vi "Convert String Data Type.vi"(5 "src byte order":T1(ring), 7 "dst byte order":T1(ring), 8 "error in (no error)":errorcluster, 9 "dst data type":T2, 10 "src data type":T2, 11 "src data in":string) -> (0 "error out":errorcluster, 3 "dst data out":string)   [LabVIEW 2019, in "DSF Core.lvlib" / "Buffer Converter.lvclass"]
uses:
  Buffer Converter.lvclass
  Typedefs/DSF Data Type.ctl
  DSF Core.lvlib
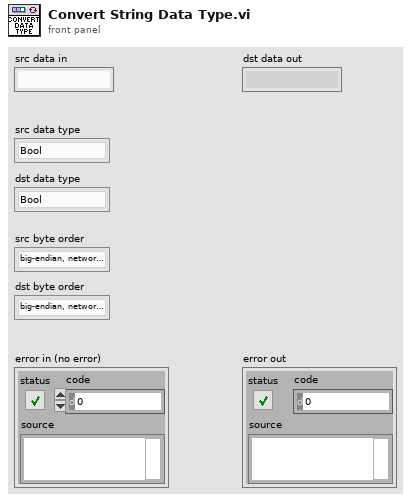
[diagram p1: front panel]
types:
  T1 = enum16{"big-endian, network order", "native, host order", "little-endian"}
  T2 = typedef "DSF Core.lvlib/DSF Data Type.ctl" = enum8{"Bool", "SGL", "DBL", "I8", "I16", "I32", "I64", "U8", "U16", "U32", "U64"}
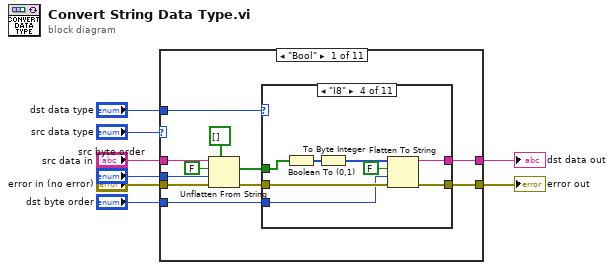
[diagram p0: block diagram]
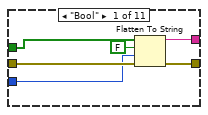
[diagram p2: hidden frame]
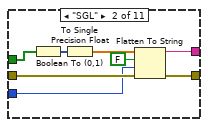
[diagram p3: hidden frame]
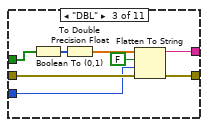
[diagram p4: hidden frame]
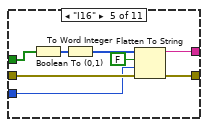
[diagram p5: hidden frame]
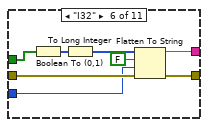
[diagram p6: hidden frame]
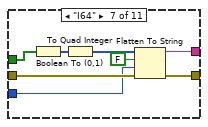
[diagram p7: hidden frame]
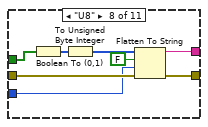
[diagram p8: hidden frame]
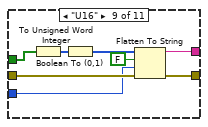
[diagram p9: hidden frame]
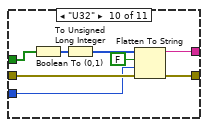
[diagram p10: hidden frame]
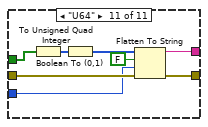
[diagram p11: hidden frame]
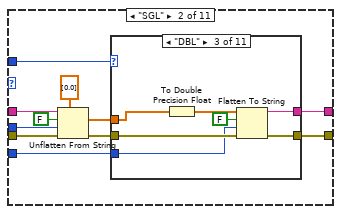
[diagram p12: hidden frame]
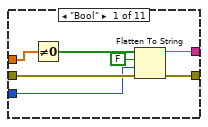
[diagram p13: hidden frame]
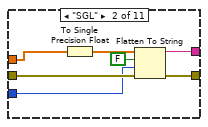
[diagram p14: hidden frame]
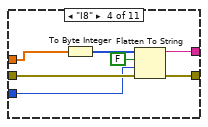
[diagram p15: hidden frame]
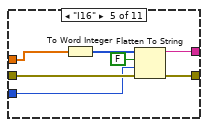
[diagram p16: hidden frame]
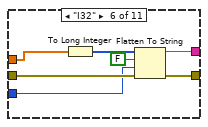
[diagram p17: hidden frame]
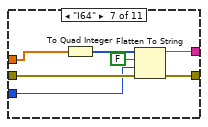
[diagram p18: hidden frame]
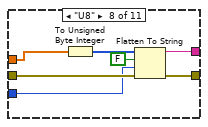
[diagram p19: hidden frame]
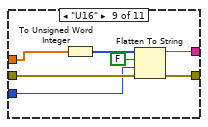
[diagram p20: hidden frame]
diagram:
  n1 = case shown="\"Bool\"" "src data type" {
    tunnel: "src data in" -> [w17 w114 w202 w290 w378 w466 w554 w642 w730 w818 w906]
    tunnel: "error in (no error)" -> [w16 w113 w201 w289 w377 w465 w553 w641 w729 w817 w905]
    tunnel: "dst data type" -> [w15 w112 w200 w288 w376 w464 w552 w640 w728 w816 w904]
    tunnel: [w12 w109 w197 w285 w373 w461 w549 w637 w725 w813 w901] -> w2
    tunnel: [w11 w108 w196 w284 w372 w460 w548 w636 w724 w812 w900] -> w8
    tunnel: "src byte order" -> [w10 w107 w195 w283 w371 w459 w547 w635 w723 w811 w899]
    tunnel: "dst byte order" -> [w9 w106 w194 w282 w370 w458 w546 w634 w722 w810 w898]
    frame "Bool" {
      n2 = Unflatten From String(type=bool[] [], binary string=w17, data includes array or string size? (T)=FALSE, byte order (0:big-endian, network order)=w10, error in (no error)=w16) -> (value=w14:bool[], error out=w13:errorcluster)  [unwired: 1 out]
      n3 = case shown="\"I8\"" w15 {
        tunnel: w14 -> [w25 w33 w41 w49 w57 w65 w73 w81 w89 w97 w105]
        tunnel: w13 -> [w24 w32 w40 w48 w56 w64 w72 w80 w88 w96 w104]
        tunnel: [w23 w31 w39 w47 w55 w63 w71 w79 w87 w95 w103] -> w12
        tunnel: [w22 w30 w38 w46 w54 w62 w70 w78 w86 w94 w102] -> w11
        tunnel: w9 -> [w21 w29 w37 w45 w53 w61 w69 w77 w85 w93 w101]
        frame "Bool" {
          n4 = Flatten To String(anything=w25, prepend array or string size? (T)=FALSE, byte order (0:big-endian, network order)=w21, error in (no error)=w24) -> (data string=w22:string, error out=w23:errorcluster)  [unwired: 1 out]
        }
        frame "SGL" {
          n5 = Boolean To (0,1)(Boolean=w33) -> (0, 1=w26:i16[])
          n6 = To Single Precision Float(number=w26) -> (single precision float=w27:sgl[])
          n7 = Flatten To String(anything=w27, prepend array or string size? (T)=FALSE, byte order (0:big-endian, network order)=w29, error in (no error)=w32) -> (data string=w30:string, error out=w31:errorcluster)  [unwired: 1 out]
        }
        frame "DBL" {
          n8 = Boolean To (0,1)(Boolean=w41) -> (0, 1=w34:i16[])
          n9 = To Double Precision Float(number=w34) -> (double precision float=w35:dbl[])
          n10 = Flatten To String(anything=w35, prepend array or string size? (T)=FALSE, byte order (0:big-endian, network order)=w37, error in (no error)=w40) -> (data string=w38:string, error out=w39:errorcluster)  [unwired: 1 out]
        }
        frame "I8" {
          n11 = Boolean To (0,1)(Boolean=w49) -> (0, 1=w42:i16[])
          n12 = To Byte Integer(number=w42) -> (8bit integer=w43:i8[])
          n13 = Flatten To String(anything=w43, prepend array or string size? (T)=FALSE, byte order (0:big-endian, network order)=w45, error in (no error)=w48) -> (data string=w46:string, error out=w47:errorcluster)  [unwired: 1 out]
        }
        frame "I16" {
          n14 = Boolean To (0,1)(Boolean=w57) -> (0, 1=w50:i16[])
          n15 = To Word Integer(number=w50) -> (16bit integer=w51:i16[])
          n16 = Flatten To String(anything=w51, prepend array or string size? (T)=FALSE, byte order (0:big-endian, network order)=w53, error in (no error)=w56) -> (data string=w54:string, error out=w55:errorcluster)  [unwired: 1 out]
        }
        frame "I32" {
          n17 = Boolean To (0,1)(Boolean=w65) -> (0, 1=w58:i16[])
          n18 = To Long Integer(number=w58) -> (32bit integer=w59:i32[])
          n19 = Flatten To String(anything=w59, prepend array or string size? (T)=FALSE, byte order (0:big-endian, network order)=w61, error in (no error)=w64) -> (data string=w62:string, error out=w63:errorcluster)  [unwired: 1 out]
        }
        frame "I64" {
          n20 = Boolean To (0,1)(Boolean=w73) -> (0, 1=w66:i16[])
          n21 = To Quad Integer(1:w66) -> (0:w67:i64[])
          n22 = Flatten To String(anything=w67, prepend array or string size? (T)=FALSE, byte order (0:big-endian, network order)=w69, error in (no error)=w72) -> (data string=w70:string, error out=w71:errorcluster)  [unwired: 1 out]
        }
        frame "U8" {
          n23 = Boolean To (0,1)(Boolean=w81) -> (0, 1=w74:i16[])
          n24 = To Unsigned Byte Integer(number=w74) -> (unsigned 8bit integer=w75:u8[])
          n25 = Flatten To String(anything=w75, prepend array or string size? (T)=FALSE, byte order (0:big-endian, network order)=w77, error in (no error)=w80) -> (data string=w78:string, error out=w79:errorcluster)  [unwired: 1 out]
        }
        frame "U16" {
          n26 = Boolean To (0,1)(Boolean=w89) -> (0, 1=w82:i16[])
          n27 = To Unsigned Word Integer(number=w82) -> (unsigned 16bit integer=w83:u16[])
          n28 = Flatten To String(anything=w83, prepend array or string size? (T)=FALSE, byte order (0:big-endian, network order)=w85, error in (no error)=w88) -> (data string=w86:string, error out=w87:errorcluster)  [unwired: 1 out]
        }
        frame "U32" {
          n29 = Boolean To (0,1)(Boolean=w97) -> (0, 1=w90:i16[])
          n30 = To Unsigned Long Integer(number=w90) -> (unsigned 32bit integer=w91:u32[])
          n31 = Flatten To String(anything=w91, prepend array or string size? (T)=FALSE, byte order (0:big-endian, network order)=w93, error in (no error)=w96) -> (data string=w94:string, error out=w95:errorcluster)  [unwired: 1 out]
        }
        frame "U64" {
          n32 = Boolean To (0,1)(Boolean=w105) -> (0, 1=w98:i16[])
          n33 = To Unsigned Quad Integer(1:w98) -> (0:w99:u64[])
          n34 = Flatten To String(anything=w99, prepend array or string size? (T)=FALSE, byte order (0:big-endian, network order)=w101, error in (no error)=w104) -> (data string=w102:string, error out=w103:errorcluster)  [unwired: 1 out]
        }
      }
    }
    frame "SGL" {
      n35 = Unflatten From String(type=sgl[] [0.0], binary string=w114, data includes array or string size? (T)=FALSE, byte order (0:big-endian, network order)=w107, error in (no error)=w113) -> (value=w111:sgl[], error out=w110:errorcluster)  [unwired: 1 out]
      n36 = case shown="\"DBL\"" w112 {
        tunnel: w111 -> [w118 w125 w132 w139 w146 w153 w160 w167 w174 w181 w188]
        tunnel: w110 -> [w123 w130 w137 w144 w151 w158 w165 w172 w179 w186 w193]
        tunnel: [w122 w129 w136 w143 w150 w157 w164 w171 w178 w185 w192] -> w109
        tunnel: [w121 w128 w135 w142 w149 w156 w163 w170 w177 w184 w191] -> w108
        tunnel: w106 -> [w120 w127 w134 w141 w148 w155 w162 w169 w176 w183 w190]
        frame "Bool" {
          n37 = Not Equal To 0?(x=w118) -> (x != 0?=w117:bool[])
          n38 = Flatten To String(anything=w117, prepend array or string size? (T)=FALSE, byte order (0:big-endian, network order)=w120, error in (no error)=w123) -> (data string=w121:string, error out=w122:errorcluster)  [unwired: 1 out]
        }
        frame "SGL" {
          n39 = To Single Precision Float(number=w125) -> (single precision float=w124:sgl[])
          n40 = Flatten To String(anything=w124, prepend array or string size? (T)=FALSE, byte order (0:big-endian, network order)=w127, error in (no error)=w130) -> (data string=w128:string, error out=w129:errorcluster)  [unwired: 1 out]
        }
        frame "DBL" {
          n41 = To Double Precision Float(number=w132) -> (double precision float=w131:dbl[])
          n42 = Flatten To String(anything=w131, prepend array or string size? (T)=FALSE, byte order (0:big-endian, network order)=w134, error in (no error)=w137) -> (data string=w135:string, error out=w136:errorcluster)  [unwired: 1 out]
        }
        frame "I8" {
          n43 = To Byte Integer(number=w139) -> (8bit integer=w138:i8[])
          n44 = Flatten To String(anything=w138, prepend array or string size? (T)=FALSE, byte order (0:big-endian, network order)=w141, error in (no error)=w144) -> (data string=w142:string, error out=w143:errorcluster)  [unwired: 1 out]
        }
        frame "I16" {
          n45 = To Word Integer(number=w146) -> (16bit integer=w145:i16[])
          n46 = Flatten To String(anything=w145, prepend array or string size? (T)=FALSE, byte order (0:big-endian, network order)=w148, error in (no error)=w151) -> (data string=w149:string, error out=w150:errorcluster)  [unwired: 1 out]
        }
        frame "I32" {
          n47 = To Long Integer(number=w153) -> (32bit integer=w152:i32[])
          n48 = Flatten To String(anything=w152, prepend array or string size? (T)=FALSE, byte order (0:big-endian, network order)=w155, error in (no error)=w158) -> (data string=w156:string, error out=w157:errorcluster)  [unwired: 1 out]
        }
        frame "I64" {
          n49 = To Quad Integer(1:w160) -> (0:w159:i64[])
          n50 = Flatten To String(anything=w159, prepend array or string size? (T)=FALSE, byte order (0:big-endian, network order)=w162, error in (no error)=w165) -> (data string=w163:string, error out=w164:errorcluster)  [unwired: 1 out]
        }
        frame "U8" {
          n51 = To Unsigned Byte Integer(number=w167) -> (unsigned 8bit integer=w166:u8[])
          n52 = Flatten To String(anything=w166, prepend array or string size? (T)=FALSE, byte order (0:big-endian, network order)=w169, error in (no error)=w172) -> (data string=w170:string, error out=w171:errorcluster)  [unwired: 1 out]
        }
        frame "U16" {
          n53 = To Unsigned Word Integer(number=w174) -> (unsigned 16bit integer=w173:u16[])
          n54 = Flatten To String(anything=w173, prepend array or string size? (T)=FALSE, byte order (0:big-endian, network order)=w176, error in (no error)=w179) -> (data string=w177:string, error out=w178:errorcluster)  [unwired: 1 out]
        }
        frame "U32" {
          n55 = To Unsigned Long Integer(number=w181) -> (unsigned 32bit integer=w180:u32[])
          n56 = Flatten To String(anything=w180, prepend array or string size? (T)=FALSE, byte order (0:big-endian, network order)=w183, error in (no error)=w186) -> (data string=w184:string, error out=w185:errorcluster)  [unwired: 1 out]
        }
        frame "U64" {
          n57 = To Unsigned Quad Integer(1:w188) -> (0:w187:u64[])
          n58 = Flatten To String(anything=w187, prepend array or string size? (T)=FALSE, byte order (0:big-endian, network order)=w190, error in (no error)=w193) -> (data string=w191:string, error out=w192:errorcluster)  [unwired: 1 out]
        }
      }
    }
    frame "DBL" {
      n59 = Unflatten From String(type=dbl[] [0.0], binary string=w202, data includes array or string size? (T)=FALSE, byte order (0:big-endian, network order)=w195, error in (no error)=w201) -> (value=w199:dbl[], error out=w198:errorcluster)  [unwired: 1 out]
      n60 = case shown="\"U64\"" w200 {
        tunnel: w199 -> [w206 w213 w220 w227 w234 w241 w248 w255 w262 w269 w276]
        tunnel: w198 -> [w211 w218 w225 w232 w239 w246 w253 w260 w267 w274 w281]
        tunnel: [w210 w217 w224 w231 w238 w245 w252 w259 w266 w273 w280] -> w197
        tunnel: [w209 w216 w223 w230 w237 w244 w251 w258 w265 w272 w279] -> w196
        tunnel: w194 -> [w208 w215 w222 w229 w236 w243 w250 w257 w264 w271 w278]
        frame "Bool" {
          n61 = Not Equal To 0?(x=w206) -> (x != 0?=w205:bool[])
          n62 = Flatten To String(anything=w205, prepend array or string size? (T)=FALSE, byte order (0:big-endian, network order)=w208, error in (no error)=w211) -> (data string=w209:string, error out=w210:errorcluster)  [unwired: 1 out]
        }
        frame "SGL" {
          n63 = To Single Precision Float(number=w213) -> (single precision float=w212:sgl[])
          n64 = Flatten To String(anything=w212, prepend array or string size? (T)=FALSE, byte order (0:big-endian, network order)=w215, error in (no error)=w218) -> (data string=w216:string, error out=w217:errorcluster)  [unwired: 1 out]
        }
        frame "DBL" {
          n65 = To Double Precision Float(number=w220) -> (double precision float=w219:dbl[])
          n66 = Flatten To String(anything=w219, prepend array or string size? (T)=FALSE, byte order (0:big-endian, network order)=w222, error in (no error)=w225) -> (data string=w223:string, error out=w224:errorcluster)  [unwired: 1 out]
        }
        frame "I8" {
          n67 = To Byte Integer(number=w227) -> (8bit integer=w226:i8[])
          n68 = Flatten To String(anything=w226, prepend array or string size? (T)=FALSE, byte order (0:big-endian, network order)=w229, error in (no error)=w232) -> (data string=w230:string, error out=w231:errorcluster)  [unwired: 1 out]
        }
        frame "I16" {
          n69 = To Word Integer(number=w234) -> (16bit integer=w233:i16[])
          n70 = Flatten To String(anything=w233, prepend array or string size? (T)=FALSE, byte order (0:big-endian, network order)=w236, error in (no error)=w239) -> (data string=w237:string, error out=w238:errorcluster)  [unwired: 1 out]
        }
        frame "I32" {
          n71 = To Long Integer(number=w241) -> (32bit integer=w240:i32[])
          n72 = Flatten To String(anything=w240, prepend array or string size? (T)=FALSE, byte order (0:big-endian, network order)=w243, error in (no error)=w246) -> (data string=w244:string, error out=w245:errorcluster)  [unwired: 1 out]
        }
        frame "I64" {
          n73 = To Quad Integer(1:w248) -> (0:w247:i64[])
          n74 = Flatten To String(anything=w247, prepend array or string size? (T)=FALSE, byte order (0:big-endian, network order)=w250, error in (no error)=w253) -> (data string=w251:string, error out=w252:errorcluster)  [unwired: 1 out]
        }
        frame "U8" {
          n75 = To Unsigned Byte Integer(number=w255) -> (unsigned 8bit integer=w254:u8[])
          n76 = Flatten To String(anything=w254, prepend array or string size? (T)=FALSE, byte order (0:big-endian, network order)=w257, error in (no error)=w260) -> (data string=w258:string, error out=w259:errorcluster)  [unwired: 1 out]
        }
        frame "U16" {
          n77 = To Unsigned Word Integer(number=w262) -> (unsigned 16bit integer=w261:u16[])
          n78 = Flatten To String(anything=w261, prepend array or string size? (T)=FALSE, byte order (0:big-endian, network order)=w264, error in (no error)=w267) -> (data string=w265:string, error out=w266:errorcluster)  [unwired: 1 out]
        }
        frame "U32" {
          n79 = To Unsigned Long Integer(number=w269) -> (unsigned 32bit integer=w268:u32[])
          n80 = Flatten To String(anything=w268, prepend array or string size? (T)=FALSE, byte order (0:big-endian, network order)=w271, error in (no error)=w274) -> (data string=w272:string, error out=w273:errorcluster)  [unwired: 1 out]
        }
        frame "U64" {
          n81 = To Unsigned Quad Integer(1:w276) -> (0:w275:u64[])
          n82 = Flatten To String(anything=w275, prepend array or string size? (T)=FALSE, byte order (0:big-endian, network order)=w278, error in (no error)=w281) -> (data string=w279:string, error out=w280:errorcluster)  [unwired: 1 out]
        }
      }
    }
    frame "I8" {
      n83 = Unflatten From String(type=i8[] [0], binary string=w290, data includes array or string size? (T)=FALSE, byte order (0:big-endian, network order)=w283, error in (no error)=w289) -> (value=w287:i8[], error out=w286:errorcluster)  [unwired: 1 out]
      n84 = case shown="\"Bool\"" w288 {
        tunnel: w287 -> [w294 w301 w308 w315 w322 w329 w336 w343 w350 w357 w364]
        tunnel: w286 -> [w299 w306 w313 w320 w327 w334 w341 w348 w355 w362 w369]
        tunnel: [w298 w305 w312 w319 w326 w333 w340 w347 w354 w361 w368] -> w285
        tunnel: [w297 w304 w311 w318 w325 w332 w339 w346 w353 w360 w367] -> w284
        tunnel: w282 -> [w296 w303 w310 w317 w324 w331 w338 w345 w352 w359 w366]
        frame "Bool" {
          n85 = Not Equal To 0?(x=w294) -> (x != 0?=w293:bool[])
          n86 = Flatten To String(anything=w293, prepend array or string size? (T)=FALSE, byte order (0:big-endian, network order)=w296, error in (no error)=w299) -> (data string=w297:string, error out=w298:errorcluster)  [unwired: 1 out]
        }
        frame "SGL" {
          n87 = To Single Precision Float(number=w301) -> (single precision float=w300:sgl[])
          n88 = Flatten To String(anything=w300, prepend array or string size? (T)=FALSE, byte order (0:big-endian, network order)=w303, error in (no error)=w306) -> (data string=w304:string, error out=w305:errorcluster)  [unwired: 1 out]
        }
        frame "DBL" {
          n89 = To Double Precision Float(number=w308) -> (double precision float=w307:dbl[])
          n90 = Flatten To String(anything=w307, prepend array or string size? (T)=FALSE, byte order (0:big-endian, network order)=w310, error in (no error)=w313) -> (data string=w311:string, error out=w312:errorcluster)  [unwired: 1 out]
        }
        frame "I8" {
          n91 = To Byte Integer(number=w315) -> (8bit integer=w314:i8[])
          n92 = Flatten To String(anything=w314, prepend array or string size? (T)=FALSE, byte order (0:big-endian, network order)=w317, error in (no error)=w320) -> (data string=w318:string, error out=w319:errorcluster)  [unwired: 1 out]
        }
        frame "I16" {
          n93 = To Word Integer(number=w322) -> (16bit integer=w321:i16[])
          n94 = Flatten To String(anything=w321, prepend array or string size? (T)=FALSE, byte order (0:big-endian, network order)=w324, error in (no error)=w327) -> (data string=w325:string, error out=w326:errorcluster)  [unwired: 1 out]
        }
        frame "I32" {
          n95 = To Long Integer(number=w329) -> (32bit integer=w328:i32[])
          n96 = Flatten To String(anything=w328, prepend array or string size? (T)=FALSE, byte order (0:big-endian, network order)=w331, error in (no error)=w334) -> (data string=w332:string, error out=w333:errorcluster)  [unwired: 1 out]
        }
        frame "I64" {
          n97 = To Quad Integer(1:w336) -> (0:w335:i64[])
          n98 = Flatten To String(anything=w335, prepend array or string size? (T)=FALSE, byte order (0:big-endian, network order)=w338, error in (no error)=w341) -> (data string=w339:string, error out=w340:errorcluster)  [unwired: 1 out]
        }
        frame "U8" {
          n99 = To Unsigned Byte Integer(number=w343) -> (unsigned 8bit integer=w342:u8[])
          n100 = Flatten To String(anything=w342, prepend array or string size? (T)=FALSE, byte order (0:big-endian, network order)=w345, error in (no error)=w348) -> (data string=w346:string, error out=w347:errorcluster)  [unwired: 1 out]
        }
        frame "U16" {
          n101 = To Unsigned Word Integer(number=w350) -> (unsigned 16bit integer=w349:u16[])
          n102 = Flatten To String(anything=w349, prepend array or string size? (T)=FALSE, byte order (0:big-endian, network order)=w352, error in (no error)=w355) -> (data string=w353:string, error out=w354:errorcluster)  [unwired: 1 out]
        }
        frame "U32" {
          n103 = To Unsigned Long Integer(number=w357) -> (unsigned 32bit integer=w356:u32[])
          n104 = Flatten To String(anything=w356, prepend array or string size? (T)=FALSE, byte order (0:big-endian, network order)=w359, error in (no error)=w362) -> (data string=w360:string, error out=w361:errorcluster)  [unwired: 1 out]
        }
        frame "U64" {
          n105 = To Unsigned Quad Integer(1:w364) -> (0:w363:u64[])
          n106 = Flatten To String(anything=w363, prepend array or string size? (T)=FALSE, byte order (0:big-endian, network order)=w366, error in (no error)=w369) -> (data string=w367:string, error out=w368:errorcluster)  [unwired: 1 out]
        }
      }
    }
    frame "I16" {
      n107 = Unflatten From String(type=i16[] [0], binary string=w378, data includes array or string size? (T)=FALSE, byte order (0:big-endian, network order)=w371, error in (no error)=w377) -> (value=w375:i16[], error out=w374:errorcluster)  [unwired: 1 out]
      n108 = case shown="\"Bool\"" w376 {
        tunnel: w375 -> [w382 w389 w396 w403 w410 w417 w424 w431 w438 w445 w452]
        tunnel: w374 -> [w387 w394 w401 w408 w415 w422 w429 w436 w443 w450 w457]
        tunnel: [w386 w393 w400 w407 w414 w421 w428 w435 w442 w449 w456] -> w373
        tunnel: [w385 w392 w399 w406 w413 w420 w427 w434 w441 w448 w455] -> w372
        tunnel: w370 -> [w384 w391 w398 w405 w412 w419 w426 w433 w440 w447 w454]
        frame "Bool" {
          n109 = Not Equal To 0?(x=w382) -> (x != 0?=w381:bool[])
          n110 = Flatten To String(anything=w381, prepend array or string size? (T)=FALSE, byte order (0:big-endian, network order)=w384, error in (no error)=w387) -> (data string=w385:string, error out=w386:errorcluster)  [unwired: 1 out]
        }
        frame "SGL" {
          n111 = To Single Precision Float(number=w389) -> (single precision float=w388:sgl[])
          n112 = Flatten To String(anything=w388, prepend array or string size? (T)=FALSE, byte order (0:big-endian, network order)=w391, error in (no error)=w394) -> (data string=w392:string, error out=w393:errorcluster)  [unwired: 1 out]
        }
        frame "DBL" {
          n113 = To Double Precision Float(number=w396) -> (double precision float=w395:dbl[])
          n114 = Flatten To String(anything=w395, prepend array or string size? (T)=FALSE, byte order (0:big-endian, network order)=w398, error in (no error)=w401) -> (data string=w399:string, error out=w400:errorcluster)  [unwired: 1 out]
        }
        frame "I8" {
          n115 = To Byte Integer(number=w403) -> (8bit integer=w402:i8[])
          n116 = Flatten To String(anything=w402, prepend array or string size? (T)=FALSE, byte order (0:big-endian, network order)=w405, error in (no error)=w408) -> (data string=w406:string, error out=w407:errorcluster)  [unwired: 1 out]
        }
        frame "I16" {
          n117 = To Word Integer(number=w410) -> (16bit integer=w409:i16[])
          n118 = Flatten To String(anything=w409, prepend array or string size? (T)=FALSE, byte order (0:big-endian, network order)=w412, error in (no error)=w415) -> (data string=w413:string, error out=w414:errorcluster)  [unwired: 1 out]
        }
        frame "I32" {
          n119 = To Long Integer(number=w417) -> (32bit integer=w416:i32[])
          n120 = Flatten To String(anything=w416, prepend array or string size? (T)=FALSE, byte order (0:big-endian, network order)=w419, error in (no error)=w422) -> (data string=w420:string, error out=w421:errorcluster)  [unwired: 1 out]
        }
        frame "I64" {
          n121 = To Quad Integer(1:w424) -> (0:w423:i64[])
          n122 = Flatten To String(anything=w423, prepend array or string size? (T)=FALSE, byte order (0:big-endian, network order)=w426, error in (no error)=w429) -> (data string=w427:string, error out=w428:errorcluster)  [unwired: 1 out]
        }
        frame "U8" {
          n123 = To Unsigned Byte Integer(number=w431) -> (unsigned 8bit integer=w430:u8[])
          n124 = Flatten To String(anything=w430, prepend array or string size? (T)=FALSE, byte order (0:big-endian, network order)=w433, error in (no error)=w436) -> (data string=w434:string, error out=w435:errorcluster)  [unwired: 1 out]
        }
        frame "U16" {
          n125 = To Unsigned Word Integer(number=w438) -> (unsigned 16bit integer=w437:u16[])
          n126 = Flatten To String(anything=w437, prepend array or string size? (T)=FALSE, byte order (0:big-endian, network order)=w440, error in (no error)=w443) -> (data string=w441:string, error out=w442:errorcluster)  [unwired: 1 out]
        }
        frame "U32" {
          n127 = To Unsigned Long Integer(number=w445) -> (unsigned 32bit integer=w444:u32[])
          n128 = Flatten To String(anything=w444, prepend array or string size? (T)=FALSE, byte order (0:big-endian, network order)=w447, error in (no error)=w450) -> (data string=w448:string, error out=w449:errorcluster)  [unwired: 1 out]
        }
        frame "U64" {
          n129 = To Unsigned Quad Integer(1:w452) -> (0:w451:u64[])
          n130 = Flatten To String(anything=w451, prepend array or string size? (T)=FALSE, byte order (0:big-endian, network order)=w454, error in (no error)=w457) -> (data string=w455:string, error out=w456:errorcluster)  [unwired: 1 out]
        }
      }
    }
    frame "I32" {
      n131 = Unflatten From String(type=i32[] [0], binary string=w466, data includes array or string size? (T)=FALSE, byte order (0:big-endian, network order)=w459, error in (no error)=w465) -> (value=w463:i32[], error out=w462:errorcluster)  [unwired: 1 out]
      n132 = case shown="\"Bool\"" w464 {
        tunnel: w463 -> [w470 w477 w484 w491 w498 w505 w512 w519 w526 w533 w540]
        tunnel: w462 -> [w475 w482 w489 w496 w503 w510 w517 w524 w531 w538 w545]
        tunnel: [w474 w481 w488 w495 w502 w509 w516 w523 w530 w537 w544] -> w461
        tunnel: [w473 w480 w487 w494 w501 w508 w515 w522 w529 w536 w543] -> w460
        tunnel: w458 -> [w472 w479 w486 w493 w500 w507 w514 w521 w528 w535 w542]
        frame "Bool" {
          n133 = Not Equal To 0?(x=w470) -> (x != 0?=w469:bool[])
          n134 = Flatten To String(anything=w469, prepend array or string size? (T)=FALSE, byte order (0:big-endian, network order)=w472, error in (no error)=w475) -> (data string=w473:string, error out=w474:errorcluster)  [unwired: 1 out]
        }
        frame "SGL" {
          n135 = To Single Precision Float(number=w477) -> (single precision float=w476:sgl[])
          n136 = Flatten To String(anything=w476, prepend array or string size? (T)=FALSE, byte order (0:big-endian, network order)=w479, error in (no error)=w482) -> (data string=w480:string, error out=w481:errorcluster)  [unwired: 1 out]
        }
        frame "DBL" {
          n137 = To Double Precision Float(number=w484) -> (double precision float=w483:dbl[])
          n138 = Flatten To String(anything=w483, prepend array or string size? (T)=FALSE, byte order (0:big-endian, network order)=w486, error in (no error)=w489) -> (data string=w487:string, error out=w488:errorcluster)  [unwired: 1 out]
        }
        frame "I8" {
          n139 = To Byte Integer(number=w491) -> (8bit integer=w490:i8[])
          n140 = Flatten To String(anything=w490, prepend array or string size? (T)=FALSE, byte order (0:big-endian, network order)=w493, error in (no error)=w496) -> (data string=w494:string, error out=w495:errorcluster)  [unwired: 1 out]
        }
        frame "I16" {
          n141 = To Word Integer(number=w498) -> (16bit integer=w497:i16[])
          n142 = Flatten To String(anything=w497, prepend array or string size? (T)=FALSE, byte order (0:big-endian, network order)=w500, error in (no error)=w503) -> (data string=w501:string, error out=w502:errorcluster)  [unwired: 1 out]
        }
        frame "I32" {
          n143 = To Long Integer(number=w505) -> (32bit integer=w504:i32[])
          n144 = Flatten To String(anything=w504, prepend array or string size? (T)=FALSE, byte order (0:big-endian, network order)=w507, error in (no error)=w510) -> (data string=w508:string, error out=w509:errorcluster)  [unwired: 1 out]
        }
        frame "I64" {
          n145 = To Quad Integer(1:w512) -> (0:w511:i64[])
          n146 = Flatten To String(anything=w511, prepend array or string size? (T)=FALSE, byte order (0:big-endian, network order)=w514, error in (no error)=w517) -> (data string=w515:string, error out=w516:errorcluster)  [unwired: 1 out]
        }
        frame "U8" {
          n147 = To Unsigned Byte Integer(number=w519) -> (unsigned 8bit integer=w518:u8[])
          n148 = Flatten To String(anything=w518, prepend array or string size? (T)=FALSE, byte order (0:big-endian, network order)=w521, error in (no error)=w524) -> (data string=w522:string, error out=w523:errorcluster)  [unwired: 1 out]
        }
        frame "U16" {
          n149 = To Unsigned Word Integer(number=w526) -> (unsigned 16bit integer=w525:u16[])
          n150 = Flatten To String(anything=w525, prepend array or string size? (T)=FALSE, byte order (0:big-endian, network order)=w528, error in (no error)=w531) -> (data string=w529:string, error out=w530:errorcluster)  [unwired: 1 out]
        }
        frame "U32" {
          n151 = To Unsigned Long Integer(number=w533) -> (unsigned 32bit integer=w532:u32[])
          n152 = Flatten To String(anything=w532, prepend array or string size? (T)=FALSE, byte order (0:big-endian, network order)=w535, error in (no error)=w538) -> (data string=w536:string, error out=w537:errorcluster)  [unwired: 1 out]
        }
        frame "U64" {
          n153 = To Unsigned Quad Integer(1:w540) -> (0:w539:u64[])
          n154 = Flatten To String(anything=w539, prepend array or string size? (T)=FALSE, byte order (0:big-endian, network order)=w542, error in (no error)=w545) -> (data string=w543:string, error out=w544:errorcluster)  [unwired: 1 out]
        }
      }
    }
    frame "I64" {
      n155 = Unflatten From String(type=i64[] [0], binary string=w554, data includes array or string size? (T)=FALSE, byte order (0:big-endian, network order)=w547, error in (no error)=w553) -> (value=w551:i64[], error out=w550:errorcluster)  [unwired: 1 out]
      n156 = case shown="\"Bool\"" w552 {
        tunnel: w551 -> [w558 w565 w572 w579 w586 w593 w600 w607 w614 w621 w628]
        tunnel: w550 -> [w563 w570 w577 w584 w591 w598 w605 w612 w619 w626 w633]
        tunnel: [w562 w569 w576 w583 w590 w597 w604 w611 w618 w625 w632] -> w549
        tunnel: [w561 w568 w575 w582 w589 w596 w603 w610 w617 w624 w631] -> w548
        tunnel: w546 -> [w560 w567 w574 w581 w588 w595 w602 w609 w616 w623 w630]
        frame "Bool" {
          n157 = Not Equal To 0?(x=w558) -> (x != 0?=w557:bool[])
          n158 = Flatten To String(anything=w557, prepend array or string size? (T)=FALSE, byte order (0:big-endian, network order)=w560, error in (no error)=w563) -> (data string=w561:string, error out=w562:errorcluster)  [unwired: 1 out]
        }
        frame "SGL" {
          n159 = To Single Precision Float(number=w565) -> (single precision float=w564:sgl[])
          n160 = Flatten To String(anything=w564, prepend array or string size? (T)=FALSE, byte order (0:big-endian, network order)=w567, error in (no error)=w570) -> (data string=w568:string, error out=w569:errorcluster)  [unwired: 1 out]
        }
        frame "DBL" {
          n161 = To Double Precision Float(number=w572) -> (double precision float=w571:dbl[])
          n162 = Flatten To String(anything=w571, prepend array or string size? (T)=FALSE, byte order (0:big-endian, network order)=w574, error in (no error)=w577) -> (data string=w575:string, error out=w576:errorcluster)  [unwired: 1 out]
        }
        frame "I8" {
          n163 = To Byte Integer(number=w579) -> (8bit integer=w578:i8[])
          n164 = Flatten To String(anything=w578, prepend array or string size? (T)=FALSE, byte order (0:big-endian, network order)=w581, error in (no error)=w584) -> (data string=w582:string, error out=w583:errorcluster)  [unwired: 1 out]
        }
        frame "I16" {
          n165 = To Word Integer(number=w586) -> (16bit integer=w585:i16[])
          n166 = Flatten To String(anything=w585, prepend array or string size? (T)=FALSE, byte order (0:big-endian, network order)=w588, error in (no error)=w591) -> (data string=w589:string, error out=w590:errorcluster)  [unwired: 1 out]
        }
        frame "I32" {
          n167 = To Long Integer(number=w593) -> (32bit integer=w592:i32[])
          n168 = Flatten To String(anything=w592, prepend array or string size? (T)=FALSE, byte order (0:big-endian, network order)=w595, error in (no error)=w598) -> (data string=w596:string, error out=w597:errorcluster)  [unwired: 1 out]
        }
        frame "I64" {
          n169 = To Quad Integer(1:w600) -> (0:w599:i64[])
          n170 = Flatten To String(anything=w599, prepend array or string size? (T)=FALSE, byte order (0:big-endian, network order)=w602, error in (no error)=w605) -> (data string=w603:string, error out=w604:errorcluster)  [unwired: 1 out]
        }
        frame "U8" {
          n171 = To Unsigned Byte Integer(number=w607) -> (unsigned 8bit integer=w606:u8[])
          n172 = Flatten To String(anything=w606, prepend array or string size? (T)=FALSE, byte order (0:big-endian, network order)=w609, error in (no error)=w612) -> (data string=w610:string, error out=w611:errorcluster)  [unwired: 1 out]
        }
        frame "U16" {
          n173 = To Unsigned Word Integer(number=w614) -> (unsigned 16bit integer=w613:u16[])
          n174 = Flatten To String(anything=w613, prepend array or string size? (T)=FALSE, byte order (0:big-endian, network order)=w616, error in (no error)=w619) -> (data string=w617:string, error out=w618:errorcluster)  [unwired: 1 out]
        }
        frame "U32" {
          n175 = To Unsigned Long Integer(number=w621) -> (unsigned 32bit integer=w620:u32[])
          n176 = Flatten To String(anything=w620, prepend array or string size? (T)=FALSE, byte order (0:big-endian, network order)=w623, error in (no error)=w626) -> (data string=w624:string, error out=w625:errorcluster)  [unwired: 1 out]
        }
        frame "U64" {
          n177 = To Unsigned Quad Integer(1:w628) -> (0:w627:u64[])
          n178 = Flatten To String(anything=w627, prepend array or string size? (T)=FALSE, byte order (0:big-endian, network order)=w630, error in (no error)=w633) -> (data string=w631:string, error out=w632:errorcluster)  [unwired: 1 out]
        }
      }
    }
    frame "U8" {
      n179 = Unflatten From String(type=u8[] [0], binary string=w642, data includes array or string size? (T)=FALSE, byte order (0:big-endian, network order)=w635, error in (no error)=w641) -> (value=w639:u8[], error out=w638:errorcluster)  [unwired: 1 out]
      n180 = case shown="\"Bool\"" w640 {
        tunnel: w639 -> [w646 w653 w660 w667 w674 w681 w688 w695 w702 w709 w716]
        tunnel: w638 -> [w651 w658 w665 w672 w679 w686 w693 w700 w707 w714 w721]
        tunnel: [w650 w657 w664 w671 w678 w685 w692 w699 w706 w713 w720] -> w637
        tunnel: [w649 w656 w663 w670 w677 w684 w691 w698 w705 w712 w719] -> w636
        tunnel: w634 -> [w648 w655 w662 w669 w676 w683 w690 w697 w704 w711 w718]
        frame "Bool" {
          n181 = Not Equal To 0?(x=w646) -> (x != 0?=w645:bool[])
          n182 = Flatten To String(anything=w645, prepend array or string size? (T)=FALSE, byte order (0:big-endian, network order)=w648, error in (no error)=w651) -> (data string=w649:string, error out=w650:errorcluster)  [unwired: 1 out]
        }
        frame "SGL" {
          n183 = To Single Precision Float(number=w653) -> (single precision float=w652:sgl[])
          n184 = Flatten To String(anything=w652, prepend array or string size? (T)=FALSE, byte order (0:big-endian, network order)=w655, error in (no error)=w658) -> (data string=w656:string, error out=w657:errorcluster)  [unwired: 1 out]
        }
        frame "DBL" {
          n185 = To Double Precision Float(number=w660) -> (double precision float=w659:dbl[])
          n186 = Flatten To String(anything=w659, prepend array or string size? (T)=FALSE, byte order (0:big-endian, network order)=w662, error in (no error)=w665) -> (data string=w663:string, error out=w664:errorcluster)  [unwired: 1 out]
        }
        frame "I8" {
          n187 = To Byte Integer(number=w667) -> (8bit integer=w666:i8[])
          n188 = Flatten To String(anything=w666, prepend array or string size? (T)=FALSE, byte order (0:big-endian, network order)=w669, error in (no error)=w672) -> (data string=w670:string, error out=w671:errorcluster)  [unwired: 1 out]
        }
        frame "I16" {
          n189 = To Word Integer(number=w674) -> (16bit integer=w673:i16[])
          n190 = Flatten To String(anything=w673, prepend array or string size? (T)=FALSE, byte order (0:big-endian, network order)=w676, error in (no error)=w679) -> (data string=w677:string, error out=w678:errorcluster)  [unwired: 1 out]
        }
        frame "I32" {
          n191 = To Long Integer(number=w681) -> (32bit integer=w680:i32[])
          n192 = Flatten To String(anything=w680, prepend array or string size? (T)=FALSE, byte order (0:big-endian, network order)=w683, error in (no error)=w686) -> (data string=w684:string, error out=w685:errorcluster)  [unwired: 1 out]
        }
        frame "I64" {
          n193 = To Quad Integer(1:w688) -> (0:w687:i64[])
          n194 = Flatten To String(anything=w687, prepend array or string size? (T)=FALSE, byte order (0:big-endian, network order)=w690, error in (no error)=w693) -> (data string=w691:string, error out=w692:errorcluster)  [unwired: 1 out]
        }
        frame "U8" {
          n195 = To Unsigned Byte Integer(number=w695) -> (unsigned 8bit integer=w694:u8[])
          n196 = Flatten To String(anything=w694, prepend array or string size? (T)=FALSE, byte order (0:big-endian, network order)=w697, error in (no error)=w700) -> (data string=w698:string, error out=w699:errorcluster)  [unwired: 1 out]
        }
        frame "U16" {
          n197 = To Unsigned Word Integer(number=w702) -> (unsigned 16bit integer=w701:u16[])
          n198 = Flatten To String(anything=w701, prepend array or string size? (T)=FALSE, byte order (0:big-endian, network order)=w704, error in (no error)=w707) -> (data string=w705:string, error out=w706:errorcluster)  [unwired: 1 out]
        }
        frame "U32" {
          n199 = To Unsigned Long Integer(number=w709) -> (unsigned 32bit integer=w708:u32[])
          n200 = Flatten To String(anything=w708, prepend array or string size? (T)=FALSE, byte order (0:big-endian, network order)=w711, error in (no error)=w714) -> (data string=w712:string, error out=w713:errorcluster)  [unwired: 1 out]
        }
        frame "U64" {
          n201 = To Unsigned Quad Integer(1:w716) -> (0:w715:u64[])
          n202 = Flatten To String(anything=w715, prepend array or string size? (T)=FALSE, byte order (0:big-endian, network order)=w718, error in (no error)=w721) -> (data string=w719:string, error out=w720:errorcluster)  [unwired: 1 out]
        }
      }
    }
    frame "U16" {
      n203 = Unflatten From String(type=u16[] [0], binary string=w730, data includes array or string size? (T)=FALSE, byte order (0:big-endian, network order)=w723, error in (no error)=w729) -> (value=w727:u16[], error out=w726:errorcluster)  [unwired: 1 out]
      n204 = case shown="\"Bool\"" w728 {
        tunnel: w727 -> [w734 w741 w748 w755 w762 w769 w776 w783 w790 w797 w804]
        tunnel: w726 -> [w739 w746 w753 w760 w767 w774 w781 w788 w795 w802 w809]
        tunnel: [w738 w745 w752 w759 w766 w773 w780 w787 w794 w801 w808] -> w725
        tunnel: [w737 w744 w751 w758 w765 w772 w779 w786 w793 w800 w807] -> w724
        tunnel: w722 -> [w736 w743 w750 w757 w764 w771 w778 w785 w792 w799 w806]
        frame "Bool" {
          n205 = Not Equal To 0?(x=w734) -> (x != 0?=w733:bool[])
          n206 = Flatten To String(anything=w733, prepend array or string size? (T)=FALSE, byte order (0:big-endian, network order)=w736, error in (no error)=w739) -> (data string=w737:string, error out=w738:errorcluster)  [unwired: 1 out]
        }
        frame "SGL" {
          n207 = To Single Precision Float(number=w741) -> (single precision float=w740:sgl[])
          n208 = Flatten To String(anything=w740, prepend array or string size? (T)=FALSE, byte order (0:big-endian, network order)=w743, error in (no error)=w746) -> (data string=w744:string, error out=w745:errorcluster)  [unwired: 1 out]
        }
        frame "DBL" {
          n209 = To Double Precision Float(number=w748) -> (double precision float=w747:dbl[])
          n210 = Flatten To String(anything=w747, prepend array or string size? (T)=FALSE, byte order (0:big-endian, network order)=w750, error in (no error)=w753) -> (data string=w751:string, error out=w752:errorcluster)  [unwired: 1 out]
        }
        frame "I8" {
          n211 = To Byte Integer(number=w755) -> (8bit integer=w754:i8[])
          n212 = Flatten To String(anything=w754, prepend array or string size? (T)=FALSE, byte order (0:big-endian, network order)=w757, error in (no error)=w760) -> (data string=w758:string, error out=w759:errorcluster)  [unwired: 1 out]
        }
        frame "I16" {
          n213 = To Word Integer(number=w762) -> (16bit integer=w761:i16[])
          n214 = Flatten To String(anything=w761, prepend array or string size? (T)=FALSE, byte order (0:big-endian, network order)=w764, error in (no error)=w767) -> (data string=w765:string, error out=w766:errorcluster)  [unwired: 1 out]
        }
        frame "I32" {
          n215 = To Long Integer(number=w769) -> (32bit integer=w768:i32[])
          n216 = Flatten To String(anything=w768, prepend array or string size? (T)=FALSE, byte order (0:big-endian, network order)=w771, error in (no error)=w774) -> (data string=w772:string, error out=w773:errorcluster)  [unwired: 1 out]
        }
        frame "I64" {
          n217 = To Quad Integer(1:w776) -> (0:w775:i64[])
          n218 = Flatten To String(anything=w775, prepend array or string size? (T)=FALSE, byte order (0:big-endian, network order)=w778, error in (no error)=w781) -> (data string=w779:string, error out=w780:errorcluster)  [unwired: 1 out]
        }
        frame "U8" {
          n219 = To Unsigned Byte Integer(number=w783) -> (unsigned 8bit integer=w782:u8[])
          n220 = Flatten To String(anything=w782, prepend array or string size? (T)=FALSE, byte order (0:big-endian, network order)=w785, error in (no error)=w788) -> (data string=w786:string, error out=w787:errorcluster)  [unwired: 1 out]
        }
        frame "U16" {
          n221 = To Unsigned Word Integer(number=w790) -> (unsigned 16bit integer=w789:u16[])
          n222 = Flatten To String(anything=w789, prepend array or string size? (T)=FALSE, byte order (0:big-endian, network order)=w792, error in (no error)=w795) -> (data string=w793:string, error out=w794:errorcluster)  [unwired: 1 out]
        }
        frame "U32" {
          n223 = To Unsigned Long Integer(number=w797) -> (unsigned 32bit integer=w796:u32[])
          n224 = Flatten To String(anything=w796, prepend array or string size? (T)=FALSE, byte order (0:big-endian, network order)=w799, error in (no error)=w802) -> (data string=w800:string, error out=w801:errorcluster)  [unwired: 1 out]
        }
        frame "U64" {
          n225 = To Unsigned Quad Integer(1:w804) -> (0:w803:u64[])
          n226 = Flatten To String(anything=w803, prepend array or string size? (T)=FALSE, byte order (0:big-endian, network order)=w806, error in (no error)=w809) -> (data string=w807:string, error out=w808:errorcluster)  [unwired: 1 out]
        }
      }
    }
    frame "U32" {
      n227 = Unflatten From String(type=u32[] [0], binary string=w818, data includes array or string size? (T)=FALSE, byte order (0:big-endian, network order)=w811, error in (no error)=w817) -> (value=w815:u32[], error out=w814:errorcluster)  [unwired: 1 out]
      n228 = case shown="\"Bool\"" w816 {
        tunnel: w815 -> [w822 w829 w836 w843 w850 w857 w864 w871 w878 w885 w892]
        tunnel: w814 -> [w827 w834 w841 w848 w855 w862 w869 w876 w883 w890 w897]
        tunnel: [w826 w833 w840 w847 w854 w861 w868 w875 w882 w889 w896] -> w813
        tunnel: [w825 w832 w839 w846 w853 w860 w867 w874 w881 w888 w895] -> w812
        tunnel: w810 -> [w824 w831 w838 w845 w852 w859 w866 w873 w880 w887 w894]
        frame "Bool" {
          n229 = Not Equal To 0?(x=w822) -> (x != 0?=w821:bool[])
          n230 = Flatten To String(anything=w821, prepend array or string size? (T)=FALSE, byte order (0:big-endian, network order)=w824, error in (no error)=w827) -> (data string=w825:string, error out=w826:errorcluster)  [unwired: 1 out]
        }
        frame "SGL" {
          n231 = To Single Precision Float(number=w829) -> (single precision float=w828:sgl[])
          n232 = Flatten To String(anything=w828, prepend array or string size? (T)=FALSE, byte order (0:big-endian, network order)=w831, error in (no error)=w834) -> (data string=w832:string, error out=w833:errorcluster)  [unwired: 1 out]
        }
        frame "DBL" {
          n233 = To Double Precision Float(number=w836) -> (double precision float=w835:dbl[])
          n234 = Flatten To String(anything=w835, prepend array or string size? (T)=FALSE, byte order (0:big-endian, network order)=w838, error in (no error)=w841) -> (data string=w839:string, error out=w840:errorcluster)  [unwired: 1 out]
        }
        frame "I8" {
          n235 = To Byte Integer(number=w843) -> (8bit integer=w842:i8[])
          n236 = Flatten To String(anything=w842, prepend array or string size? (T)=FALSE, byte order (0:big-endian, network order)=w845, error in (no error)=w848) -> (data string=w846:string, error out=w847:errorcluster)  [unwired: 1 out]
        }
        frame "I16" {
          n237 = To Word Integer(number=w850) -> (16bit integer=w849:i16[])
          n238 = Flatten To String(anything=w849, prepend array or string size? (T)=FALSE, byte order (0:big-endian, network order)=w852, error in (no error)=w855) -> (data string=w853:string, error out=w854:errorcluster)  [unwired: 1 out]
        }
        frame "I32" {
          n239 = To Long Integer(number=w857) -> (32bit integer=w856:i32[])
          n240 = Flatten To String(anything=w856, prepend array or string size? (T)=FALSE, byte order (0:big-endian, network order)=w859, error in (no error)=w862) -> (data string=w860:string, error out=w861:errorcluster)  [unwired: 1 out]
        }
        frame "I64" {
          n241 = To Quad Integer(1:w864) -> (0:w863:i64[])
          n242 = Flatten To String(anything=w863, prepend array or string size? (T)=FALSE, byte order (0:big-endian, network order)=w866, error in (no error)=w869) -> (data string=w867:string, error out=w868:errorcluster)  [unwired: 1 out]
        }
        frame "U8" {
          n243 = To Unsigned Byte Integer(number=w871) -> (unsigned 8bit integer=w870:u8[])
          n244 = Flatten To String(anything=w870, prepend array or string size? (T)=FALSE, byte order (0:big-endian, network order)=w873, error in (no error)=w876) -> (data string=w874:string, error out=w875:errorcluster)  [unwired: 1 out]
        }
        frame "U16" {
          n245 = To Unsigned Word Integer(number=w878) -> (unsigned 16bit integer=w877:u16[])
          n246 = Flatten To String(anything=w877, prepend array or string size? (T)=FALSE, byte order (0:big-endian, network order)=w880, error in (no error)=w883) -> (data string=w881:string, error out=w882:errorcluster)  [unwired: 1 out]
        }
        frame "U32" {
          n247 = To Unsigned Long Integer(number=w885) -> (unsigned 32bit integer=w884:u32[])
          n248 = Flatten To String(anything=w884, prepend array or string size? (T)=FALSE, byte order (0:big-endian, network order)=w887, error in (no error)=w890) -> (data string=w888:string, error out=w889:errorcluster)  [unwired: 1 out]
        }
        frame "U64" {
          n249 = To Unsigned Quad Integer(1:w892) -> (0:w891:u64[])
          n250 = Flatten To String(anything=w891, prepend array or string size? (T)=FALSE, byte order (0:big-endian, network order)=w894, error in (no error)=w897) -> (data string=w895:string, error out=w896:errorcluster)  [unwired: 1 out]
        }
      }
    }
    frame "U64" {
      n251 = Unflatten From String(type=u64[] [0], binary string=w906, data includes array or string size? (T)=FALSE, byte order (0:big-endian, network order)=w899, error in (no error)=w905) -> (value=w903:u64[], error out=w902:errorcluster)  [unwired: 1 out]
      n252 = case shown="\"Bool\"" w904 {
        tunnel: w903 -> [w910 w917 w924 w931 w938 w945 w952 w959 w966 w973 w980]
        tunnel: w902 -> [w915 w922 w929 w936 w943 w950 w957 w964 w971 w978 w985]
        tunnel: [w914 w921 w928 w935 w942 w949 w956 w963 w970 w977 w984] -> w901
        tunnel: [w913 w920 w927 w934 w941 w948 w955 w962 w969 w976 w983] -> w900
        tunnel: w898 -> [w912 w919 w926 w933 w940 w947 w954 w961 w968 w975 w982]
        frame "Bool" {
          n253 = Not Equal To 0?(x=w910) -> (x != 0?=w909:bool[])
          n254 = Flatten To String(anything=w909, prepend array or string size? (T)=FALSE, byte order (0:big-endian, network order)=w912, error in (no error)=w915) -> (data string=w913:string, error out=w914:errorcluster)  [unwired: 1 out]
        }
        frame "SGL" {
          n255 = To Single Precision Float(number=w917) -> (single precision float=w916:sgl[])
          n256 = Flatten To String(anything=w916, prepend array or string size? (T)=FALSE, byte order (0:big-endian, network order)=w919, error in (no error)=w922) -> (data string=w920:string, error out=w921:errorcluster)  [unwired: 1 out]
        }
        frame "DBL" {
          n257 = To Double Precision Float(number=w924) -> (double precision float=w923:dbl[])
          n258 = Flatten To String(anything=w923, prepend array or string size? (T)=FALSE, byte order (0:big-endian, network order)=w926, error in (no error)=w929) -> (data string=w927:string, error out=w928:errorcluster)  [unwired: 1 out]
        }
        frame "I8" {
          n259 = To Byte Integer(number=w931) -> (8bit integer=w930:i8[])
          n260 = Flatten To String(anything=w930, prepend array or string size? (T)=FALSE, byte order (0:big-endian, network order)=w933, error in (no error)=w936) -> (data string=w934:string, error out=w935:errorcluster)  [unwired: 1 out]
        }
        frame "I16" {
          n261 = To Word Integer(number=w938) -> (16bit integer=w937:i16[])
          n262 = Flatten To String(anything=w937, prepend array or string size? (T)=FALSE, byte order (0:big-endian, network order)=w940, error in (no error)=w943) -> (data string=w941:string, error out=w942:errorcluster)  [unwired: 1 out]
        }
        frame "I32" {
          n263 = To Long Integer(number=w945) -> (32bit integer=w944:i32[])
          n264 = Flatten To String(anything=w944, prepend array or string size? (T)=FALSE, byte order (0:big-endian, network order)=w947, error in (no error)=w950) -> (data string=w948:string, error out=w949:errorcluster)  [unwired: 1 out]
        }
        frame "I64" {
          n265 = To Quad Integer(1:w952) -> (0:w951:i64[])
          n266 = Flatten To String(anything=w951, prepend array or string size? (T)=FALSE, byte order (0:big-endian, network order)=w954, error in (no error)=w957) -> (data string=w955:string, error out=w956:errorcluster)  [unwired: 1 out]
        }
        frame "U8" {
          n267 = To Unsigned Byte Integer(number=w959) -> (unsigned 8bit integer=w958:u8[])
          n268 = Flatten To String(anything=w958, prepend array or string size? (T)=FALSE, byte order (0:big-endian, network order)=w961, error in (no error)=w964) -> (data string=w962:string, error out=w963:errorcluster)  [unwired: 1 out]
        }
        frame "U16" {
          n269 = To Unsigned Word Integer(number=w966) -> (unsigned 16bit integer=w965:u16[])
          n270 = Flatten To String(anything=w965, prepend array or string size? (T)=FALSE, byte order (0:big-endian, network order)=w968, error in (no error)=w971) -> (data string=w969:string, error out=w970:errorcluster)  [unwired: 1 out]
        }
        frame "U32" {
          n271 = To Unsigned Long Integer(number=w973) -> (unsigned 32bit integer=w972:u32[])
          n272 = Flatten To String(anything=w972, prepend array or string size? (T)=FALSE, byte order (0:big-endian, network order)=w975, error in (no error)=w978) -> (data string=w976:string, error out=w977:errorcluster)  [unwired: 1 out]
        }
        frame "U64" {
          n273 = To Unsigned Quad Integer(1:w980) -> (0:w979:u64[])
          n274 = Flatten To String(anything=w979, prepend array or string size? (T)=FALSE, byte order (0:big-endian, network order)=w982, error in (no error)=w985) -> (data string=w983:string, error out=w984:errorcluster)  [unwired: 1 out]
        }
      }
    }
  }
  "dst data out" <- w8
  "error out" <- w2
